vi "configure.vi"(8 "error in (no error)":errorcluster, 11 "ILCSim1TC in":refnum<class "ILCSim1TC.lvclass">) -> (0 "error out":errorcluster, 3 "ILCSim1TC out":refnum<class "ILCSim1TC.lvclass">)   [LabVIEW 2015, in "ILCSim1TC.lvclass"]
uses:
  ILCSim1TC.lvclass
  <userlib>/Common/ILC/Configuration/ADC Collection Settings.ctl
  <userlib>/Common/ILC/Typedefs/Input Channels.ctl
  <userlib>/Common/ILC/Typedefs/Scan Rates.ctl
  <userlib>/Common/Simulators/ILCSim1/ILCSim1.lvclass/ILCSim1.ctl
  ConfigurationThisComponent/ConfigurationThisComponent.lvclass
  <userlib>/Common/Simulators/ILCSim1/ILCSim1.lvclass
  <userlib>/Common/ILC/Typedefs/ILCTypedefs.lvlib
  <userlib>/Common/ILC/Configuration/ILCConfiguration.lvlib
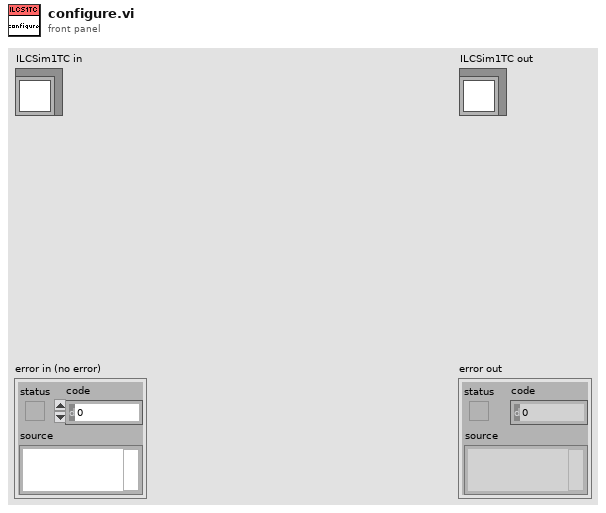
[diagram p1: front panel]
types:
  T1 = typedef "ILCCommon.lvlib/ILCConfiguration.lvlib/ADC Collection Settings.ctl" = cluster{"Input Channels":T2, "Scan Rate (Hz) ":T3, "PGA Gain Coefficient":u8}
  T2 = typedef "ILCCommon.lvlib/ILCTypedefs.lvlib/Input Channels.ctl" = enum16{"Channel 0", "3 Channels", "5 Channels"}
  T3 = typedef "ILCCommon.lvlib/ILCTypedefs.lvlib/Scan Rates.ctl" = enum16{"50", "60", "100", "120", "200", "240", "300", "400", "480", "600", "1200", "2400", "4800"}
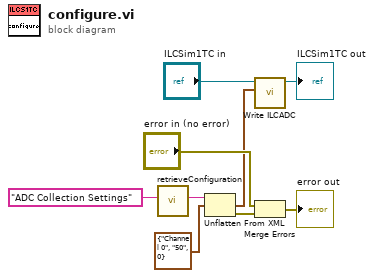
[diagram p0: block diagram]
diagram:
  n1 = call "retrieveConfiguration.vi"("configName"="ADC Collection Settings") -> ("xmlConfig"=w8:string)  [unwired: 8 in, 2 out]
  n2 = Unflatten From XML(xml string=w8, type=T1 {"Input Channels"=enum."Channel 0", "Scan Rate (Hz) "=enum."50", "PGA Gain Coefficient"=0} ("ADC Settings")) -> (value=w3:T1, error out=w7:errorcluster)  [unwired: 1 in]
  n3 = call <userlib>:"Write ILCADC.vi"("ADC Collection Settings"=w3, "ILCSim1 in"="ILCSim1TC in") -> ("ILCSim1 out"=→"ILCSim1TC out":refnum<class "ILCSim1TC.lvclass">)  [unwired: 9 in]
  n4 = Merge Errors("error in (no error)", w7) -> (→"error out":errorcluster)
